vi "fgv_remote_conn-check.vi"(7 "cmd":enum16{"write", "read"}(ring), 11 "conn":bool) -> (3 "conn_result":bool)   [LabVIEW 2019]
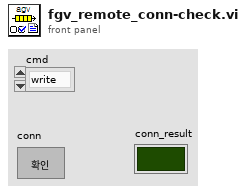
[diagram p1: front panel]
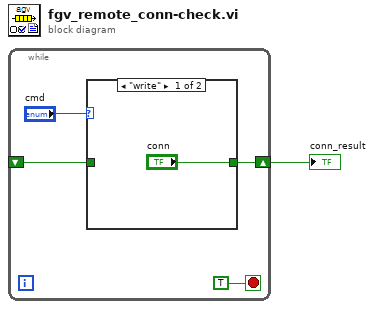
[diagram p0: block diagram]
diagram:
  n1 = while {
    shift-right: [w3] -> w1
    shift-left: _ -> [w2]
    stop <- TRUE stop-if-true
    n2 = case shown="\"write\"" "cmd" {
      tunnel: ["conn" w7] -> w3
      tunnel: w2 -> [_ w7]
      frame "write" {
      }
      frame "read", Default {
      }
    }
  }
  "conn_result" <- w1
